vi "Start Test.vi"(8 "error in (no error)":errorcluster, 10 "Tests":string[](array[string]), 11 "XML Report in":refnum<class "Report.lvclass">) -> (0 "error out":errorcluster, 3 "XML Report out":refnum<class "Report.lvclass">)   [LabVIEW 2020, in "Reports.lvlib" / "Report.lvclass"]
uses:
  Report.lvclass
  Report.lvclass/Report.ctl
  Report Generator/Report Generator.lvclass
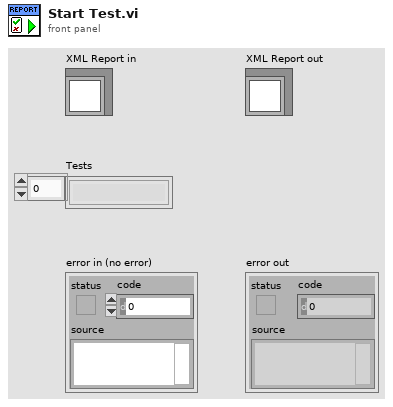
[diagram p1: front panel]
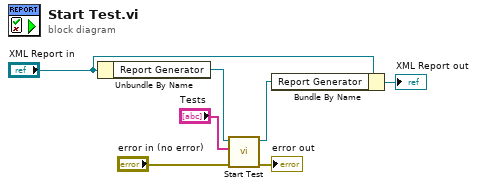
[diagram p0: block diagram]
diagram:
  n1 = Unbundle By Name("XML Report in") -> ("Report Generator"=w7:refnum<class "Report Generator.lvclass">)
  n2 = call-dynamic "Start Test.vi"("error in (no error)"="error in (no error)", "Tests"="Tests", "Report Generator In"=w7) -> ("error out"=→"error out":errorcluster, "Report Generator Out"=w2:refnum<class "Report Generator.lvclass">)  [unwired: 7 in]
  n3 = Bundle By Name(cluster="XML Report in", "Report Generator"=w2) -> (→"XML Report out":refnum<class "Report.lvclass">)
